vi "CreateFrequencyArray.vi"(10 "Signal":dbl[](array[numeric]), 11 "Actual Sampling rate (Hz)":dbl) -> (3 "Frequencies":dbl[](array[numeric]))   [LabVIEW 2011]
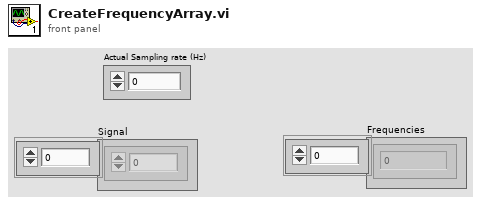
[diagram p1: front panel]
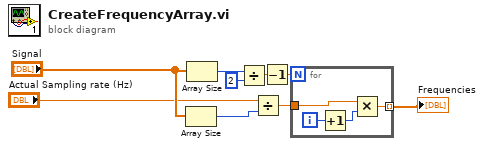
[diagram p0: block diagram]
diagram:
  n1 = Array Size(array="Signal") -> (size(s)=w3:i32)
  n2 = Array Size(array="Signal") -> (size(s)=w6:i32)
  n3 = Divide(x=w6, y=2) -> (x/y=w8:dbl)
  n4 = Divide(x="Actual Sampling rate (Hz)", y=w3) -> (x/y=w2:dbl)
  n5 = Decrement(x=w8) -> (x-1=w9:dbl)
  n6 = for {
    N: w9 -> [_]
    tunnel: w2 -> [w11]
    tunnel: [w10] -> w4 mode=indexing
    i -> [w13]
    n7 = Increment(x=w13) -> (x+1=w12:i32)
    n8 = Multiply(x=w11, y=w12) -> (x*y=w10:dbl)
  }
  "Frequencies" <- w4
